vi "WSVCAP SHL FPGA LL Procedure I2C - Receive Byte.vi"(0 "Procedure Step":T1, 1 "Wait Ticks Remaining":u32, 5 "I2C Wait Ticks":u32, 7 "Read Bits Remaining":u8, 9 "Read Bytes Remaining":u8, 11 "error in (no error)":errorcluster, 13 "Socket Mask":u64 format="%012x", 14 "UUT Set (0/1)":u8) -> (3 "Wait Ticks Remaining Out":u32, 4 "Procedure Step Out":T1, 6 "Finished":bool, 8 "Read Bits Remaining Out":u8, 10 "Read Bytes Remaining Out":u8, 15 "error out":errorcluster)   [LabVIEW 2012]
uses:
  Type Defs/WSVCAP SHL Procedure Step Enum.ctl
  Type Defs/WSVCAP SHL I2C Write Line Enum.ctl
  Type Defs/WSVCAP SHL FIFO Operation Enum.ctl
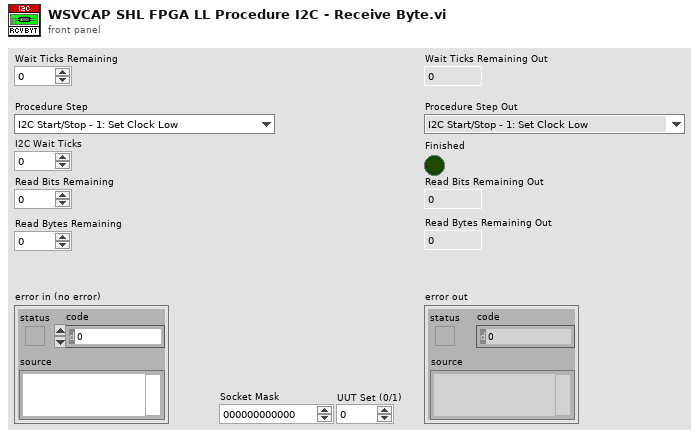
[diagram p1: front panel]
types:
  T1 = typedef "WSVCAP SHL Procedure Step Enum.ctl" = enum16{"I2C Start/Stop - 1: Set Clock Low", "I2C Start/Stop - 2: Wait", "I2C Start/Stop - 3: Set Data I", "I2C Start/Stop - 4: Wait", "I2C Start/Stop - 5: Set Clock High", "I2C Start/Stop - 6: Wait", "I2C Start/Stop - 7: Set Data II", "I2C Start/Stop - 8: Wait", "I2C Start/Stop - 9: Set Clock Low", "I2C Start/Stop - 10: Wait", "I2C Read ACK - 1: Set Clock High", "I2C Read ACK - 2: Wait", "I2C Read ACK - 3: Read ACK Bit", "I2C Read ACK - 4: Wait", "I2C Read ACK - 5: Set Clock Low", "I2C Read ACK - 6: Wait", "I2C Write ACK - 1: Write ACK Bit", "I2C Write ACK - 2: Wait", "I2C Write ACK - 3: Set Clock High", "I2C Write ACK - 4: Wait", "I2C Write ACK - 5: Set Clock Low", "I2C Write ACK - 6: Wait", "I2C Write ACK - 7: Set Data Low", "I2C Send Add - 1: Reset Bits Remaining", "I2C Send Add - 2: Set Data Bit", "I2C Send Add - 3: Wait", "I2C Send Add - 4: Set Clock High", "I2C Send Add - 5: Wait", "I2C Send Add - 6: Set Clock Low", "I2C Send Add - 7: Wait", "I2C Send Add - 8: Check Bits Remaining", "I2C Send Data - 1: Reset Bits Remaining", "I2C Send Data - 2: Load Write Bit from FIFO", "I2C Send Data - 3: Set Data Bit", "I2C Send Data - 4: Wait", "I2C Send Data - 5: Set Clock High", "I2C Send Data - 6: Wait", "I2C Send Data - 7: Set Clock Low", "I2C Send Data - 8: Wait", "I2C Send Data - 9: Check Bits Remaining", "I2C Receive Data - 1: Reset Bits Remaining", "I2C Receive Data - 2: Wait", "I2C Receive Data - 3: Set Clock High", "I2C Receive Data - 4: Wait", "I2C Receive Data - 5: Read Data Bit", "I2C Receive Data - 6: Wait", "I2C Receive Data - 7: Set Clock Low", "I2C Receive Data - 8: Wait", "I2C Receive Data - 9: Check Bits Remaining", "RFFE Send SSC - 1:Set Low", "RFFE Send SSC - 2:Wait", "RFFE Send SSC - 3:Set SDA High", "RFFE Send SSC - 4:Wait", "RFFE Send SSC - 5:Set SDA Low", "RFFE Send SSC - 6:Wait", "RFFE Send Data - 1:Set SCL High", "RFFE Send Data - 2:Wait", "RFFE Send Data - 3:Set SCL Low", "RFFE Send Data - 4:Wait", "RFFE Send Data - 5:Set SCL High (P)", "RFFE Send Data - 6:Wait", "RFFE Send Data - 7:Set SCL Low (P)", "RFFE Send Data - 8:Wait", "RFFE Send Data - 9:Set SCL High (BP)", "RFFE Send Data - 10:Wait", "RFFE Send Data - 11:Set SCL Low (BP)", "RFFE Send Data - 12:Wait", "RFFE Receive Data - 1:Set SCL High", "RFFE Receive Data - 2:Wait", "RFFE Receive Data - 3:Set SCL Low", "RFFE Receive Data - 4:Wait", "RFFE Receive Data - 5:Set SCL High (BP)", "RFFE Receive Data - 6:Wait", "RFFE Receive Data - 7:Set SCL Low (BP)", "RFFE Receive Data - 8:Wait", "RFFE Wait CMD Delay - 1:Wait", "RFFE Clear Lines - 1:Clear"}
  T2 = typedef "WSVCAP SHL I2C Write Line Enum.ctl" = enum16{"I2C SCL", "I2C SDA"}
  T3 = typedef "WSVCAP SHL FIFO Operation Enum.ctl" = enum16{"Create FIFO/Memory", "Get Write FIFO Status", "Get Read FIFO Status", "Put Element in Write", "Put Element in Read", "Get Element from Write", "Get Element from Read"}
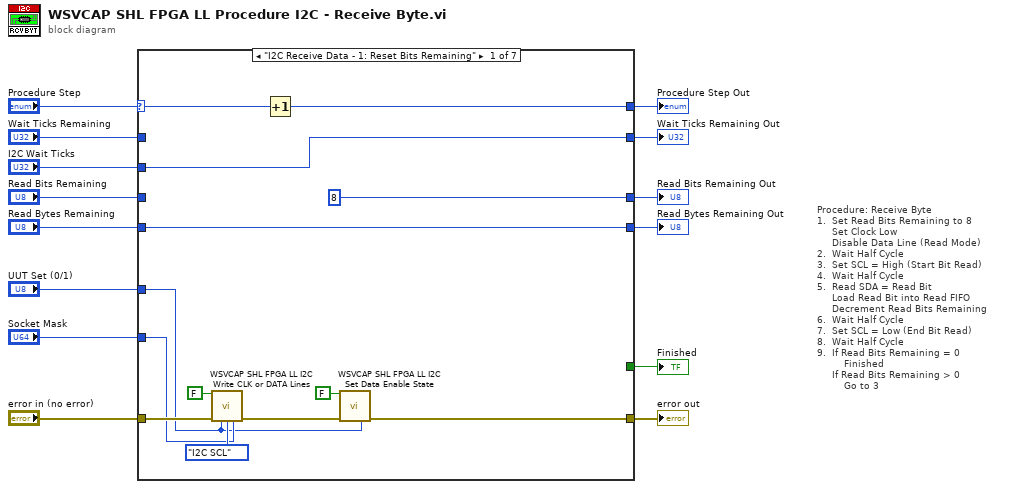
[diagram p0: block diagram]
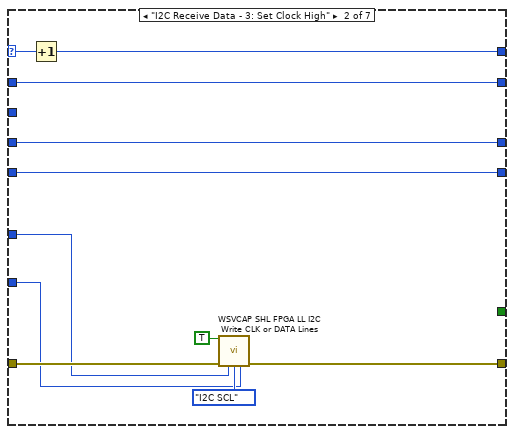
[diagram p2: hidden frame]
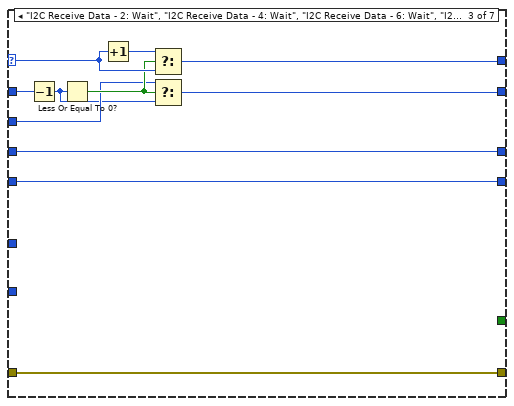
[diagram p3: hidden frame]
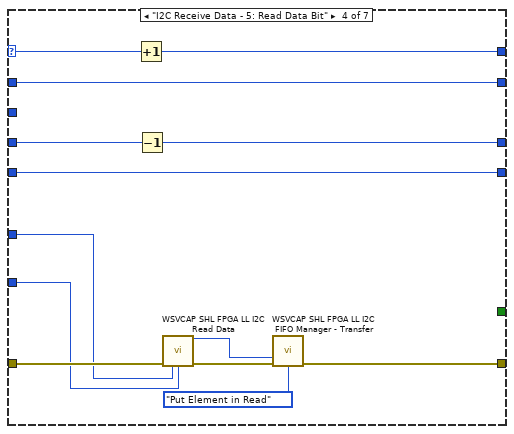
[diagram p4: hidden frame]
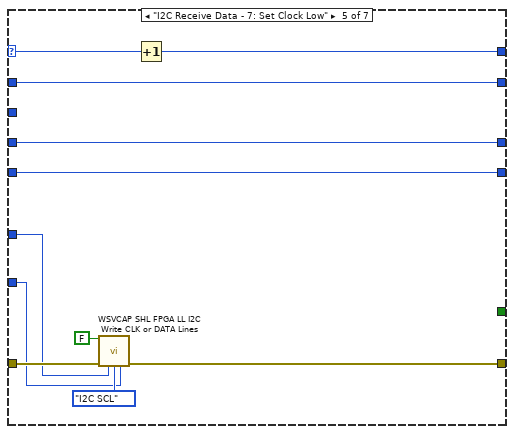
[diagram p5: hidden frame]
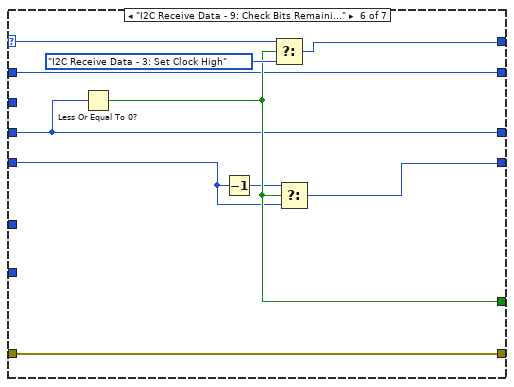
[diagram p6: hidden frame]
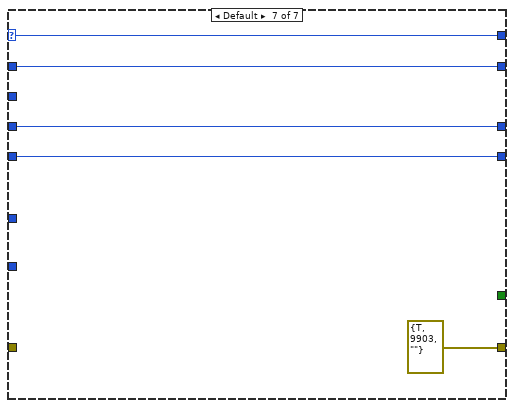
[diagram p7: hidden frame]
diagram:
  # "Procedure: Receive Byte\n1.  Set Read Bits Remaining to 8 \n     Set Clock Low\n     Disable Data Line (Read Mode)\n2.  Wait Half Cycle\n3.  Set SCL = High (Start Bit Read)\n4.  Wait Half Cycle\n5.  Read SDA = Read Bit\n     Load Read Bit into Read FIFO\n     Decrement Read Bits Remaining\n6.  Wait Half Cycle\n7.  Set SCL = Low (End Bit Read)\n8.  Wait Half Cycle\n9.  If Read Bits Remaining = 0\n         Finished\n     If Read Bits Remaining > 0\n         Go to 3"
  n1 = case shown="\"I2C Receive Data - 1: Reset Bits Remaining\"" "Procedure Step" {
    selector: "Procedure Step" -> [w24 w35 w48 w61 w69 w78 w87]
    tunnel: [w22 w36 w46 w59 w71 w83 errorcluster {"status"=TRUE, "code"=9903, "source"=""} ("error IO")] -> w13
    tunnel: "error in (no error)" -> [w26 w37 w46 w62 w72 w83 _]
    tunnel: "Wait Ticks Remaining" -> [_ w31 w49 w52 w66 w75 w86]
    tunnel: "I2C Wait Ticks" -> [w17 _ w44 _ _ _ _]
    tunnel: "Read Bits Remaining" -> [_ w30 w40 w56 w65 w74 w85]
    tunnel: [_ _ _ _ _ w81 _] -> w12
    tunnel: "Socket Mask" -> [w20 w33 _ w55 w68 _ _]
    tunnel: "Read Bytes Remaining" -> [w16 w29 w39 w51 w64 w80 w84]
    tunnel: [w19 w32 w42 w54 w67 w77 w87] -> w11
    tunnel: [w16 w29 w39 w51 w64 w76 w84] -> w10
    tunnel: [w17 w31 w41 w52 w66 w75 w86] -> w3
    tunnel: [u8 8 ("Write Bits Remaining") w30 w40 w53 w65 w74 w85] -> w2
    tunnel: "UUT Set (0/1)" -> [w15 w28 _ w50 w63 _ _]
    frame "I2C Receive Data - 1: Reset Bits Remaining" {
      n2 = call "WSVCAP SHL FPGA LL I2C Write CLK or DATA Lines.vi"("Bit In"=FALSE, "error in (no error)"=w26, "UUT Set (0/1)"=w15, "Line"=WSVCAP_SHL_I2C_Write_Line_Enum."I2C SCL", "Socket Mask"=w20) -> ("error out"=w23:errorcluster)  [unwired: 10 in]
      n3 = Increment(x=w24) -> (x+1=w19:T1)
      n4 = call "WSVCAP SHL FPGA LL I2C Set Data Enable State.vi"("State"=FALSE, "error in (no error)"=w23, "UUT Set (0/1)"=w15) -> ("error out"=w22:errorcluster)  [unwired: 12 in]
    }
    frame "I2C Receive Data - 3: Set Clock High" {
      n5 = Increment(x=w35) -> (x+1=w32:T1)
      n6 = call "WSVCAP SHL FPGA LL I2C Write CLK or DATA Lines.vi"("Bit In"=TRUE, "error in (no error)"=w37, "UUT Set (0/1)"=w28, "Line"=WSVCAP_SHL_I2C_Write_Line_Enum."I2C SCL", "Socket Mask"=w33) -> ("error out"=w36:errorcluster)  [unwired: 10 in]
    }
    frame "I2C Receive Data - 2: Wait", "I2C Receive Data - 4: Wait", "I2C Receive Data - 6: Wait", "I2C Receive Data - 8: Wait" {
      n7 = Decrement(x=w49) -> (x-1=w43:u32)
      n8 = Less Or Equal To 0?(x=w43) -> (x <= 0?=w45:bool)
      n9 = Increment(x=w48) -> (x+1=w47:T1)
      n10 = Select(t=w47, s=w45, f=w48) -> (s? t:f=w42:T1)
      n11 = Select(t=w44, s=w45, f=w43) -> (s? t:f=w41:u32)
    }
    frame "I2C Receive Data - 5: Read Data Bit" {
      n12 = Increment(x=w61) -> (x+1=w54:T1)
      n13 = Decrement(x=w56) -> (x-1=w53:u8)
      n14 = call "WSVCAP SHL FPGA LL I2C Read Data.vi"("error in (no error)"=w62, "UUT Set (0-1)"=w50, "Socket Mask"=w55) -> ("Long Word Out (1-Bit for Each Channel)"=w57:u64, "error out"=w60:errorcluster)  [unwired: 11 in]
      n15 = call "WSVCAP SHL FPGA LL I2C FIFO Manager - Transfer.vi"("Long Word In"=w57, "error in (no error)"=w60, "Operation"=WSVCAP_SHL_FIFO_Operation_Enum."Put Element in Read") -> ("error out"=w59:errorcluster)  [unwired: 10 in, 2 out]
    }
    frame "I2C Receive Data - 7: Set Clock Low" {
      n16 = call "WSVCAP SHL FPGA LL I2C Write CLK or DATA Lines.vi"("Bit In"=FALSE, "error in (no error)"=w72, "UUT Set (0/1)"=w63, "Line"=WSVCAP_SHL_I2C_Write_Line_Enum."I2C SCL", "Socket Mask"=w68) -> ("error out"=w71:errorcluster)  [unwired: 10 in]
      n17 = Increment(x=w69) -> (x+1=w67:T1)
    }
    frame "I2C Receive Data - 9: Check Bits Remaining" {
      n18 = Less Or Equal To 0?(x=w74) -> (x <= 0?=w81:bool)
      n19 = Decrement(x=w80) -> (x-1=w79:u8)
      n20 = Select(t=w78, s=w81, f=WSVCAP_SHL_Procedure_Step_Enum."I2C Receive Data - 3: Set Clock High" ("Procedure Step")) -> (s? t:f=w77:T1)
      n21 = Select(t=w79, s=w81, f=w80) -> (s? t:f=w76:u8)
    }
    frame Default {
    }
  }
  "error out" <- w13
  "Finished" <- w12
  "Procedure Step Out" <- w11
  "Read Bytes Remaining Out" <- w10
  "Wait Ticks Remaining Out" <- w3
  "Read Bits Remaining Out" <- w2
